vi "Resistive card.vi"(8 "error in (no error)":errorcluster, 11 "Node Ptr":T2 format="%.0x") -> (0 "error out":errorcluster)   [LabVIEW 2014, in "SLSC configuration System Explorer.lvlib"]
uses:
  SLSC configuration System Explorer.lvlib
  <vilib>/NI Veristand/Custom Device API/Custom Device Item Ref.ctl
  Shared/Card Postion.ctl
  Shared/Constants.vi
  <vilib>/NI Veristand/Custom Device API/Get Item Property (U16).vi
  <vilib>/NI Veristand/Custom Device API/Set Item Property (Variant).vi
  <vilib>/NI Veristand/Custom Device API/Custom Device API.lvlib
  Shared/SLSC configuration Shared.lvlib
panel:
  in  "Card Position":T1
  in  "CH 7 (ohms)":dbl min=0.0 max=8191.875 step=0.125 format="%#_7g"
  in  "CH 6 (ohms)":dbl min=0.0 max=8191.875 step=0.125 format="%#_7g"
  in  "CH 5 (ohms)":dbl min=0.0 max=8191.875 step=0.125 format="%#_7g"
  in  "CH 4 (ohms)":dbl min=0.0 max=8191.875 step=0.125 format="%#_7g"
  in  "CH 3(ohms)":dbl min=0.0 max=8191.875 step=0.125 format="%#_7g"
  in  "CH 2 (ohms)":dbl min=0.0 max=8191.875 step=0.125 format="%#_7g"
  in  "CH 1(ohms)":dbl min=0.0 max=8191.875 step=0.125 format="%#_7g"
  in  "Header 2":cluster{"Section Name":string}={"Section Name"="FIU Initial Configuration"}
  in  "CH 0 (ohms)":dbl min=0.0 max=8191.875 step=0.125 format="%#_7g"
  in  "Header":cluster{"Section Name":string}={"Section Name"="FIU Card Settings"}
  in  "Description":string
  in  "Name":string
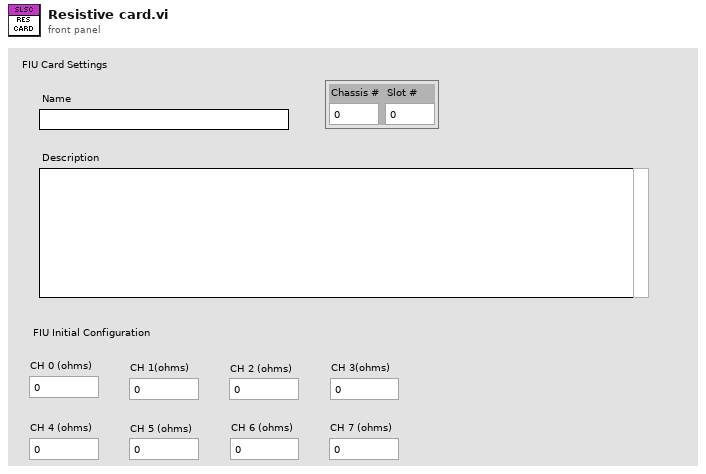
[diagram p1: front panel]
types:
  T1 = typedef "SLSC configuration Shared.lvlib/Card Postion.ctl" = cluster{"Chassis #":u8, "Slot #":u8}
  T2 = typedef "Custom Device API.lvlib/Custom Device Item Ref.ctl" = u64
  T3 = typedef "Custom Device API.lvlib/Custom Device Commands.ctl" = enum16{"Default", "Item renamed", "Shutdown", "Dynamic button pressed"}
  T4 = typedef "Custom Device API.lvlib/Custom Device Item Info.ctl" = cluster{"Name":string, "Is Channel":bool, "GUID":string, "Is Waveform":bool}
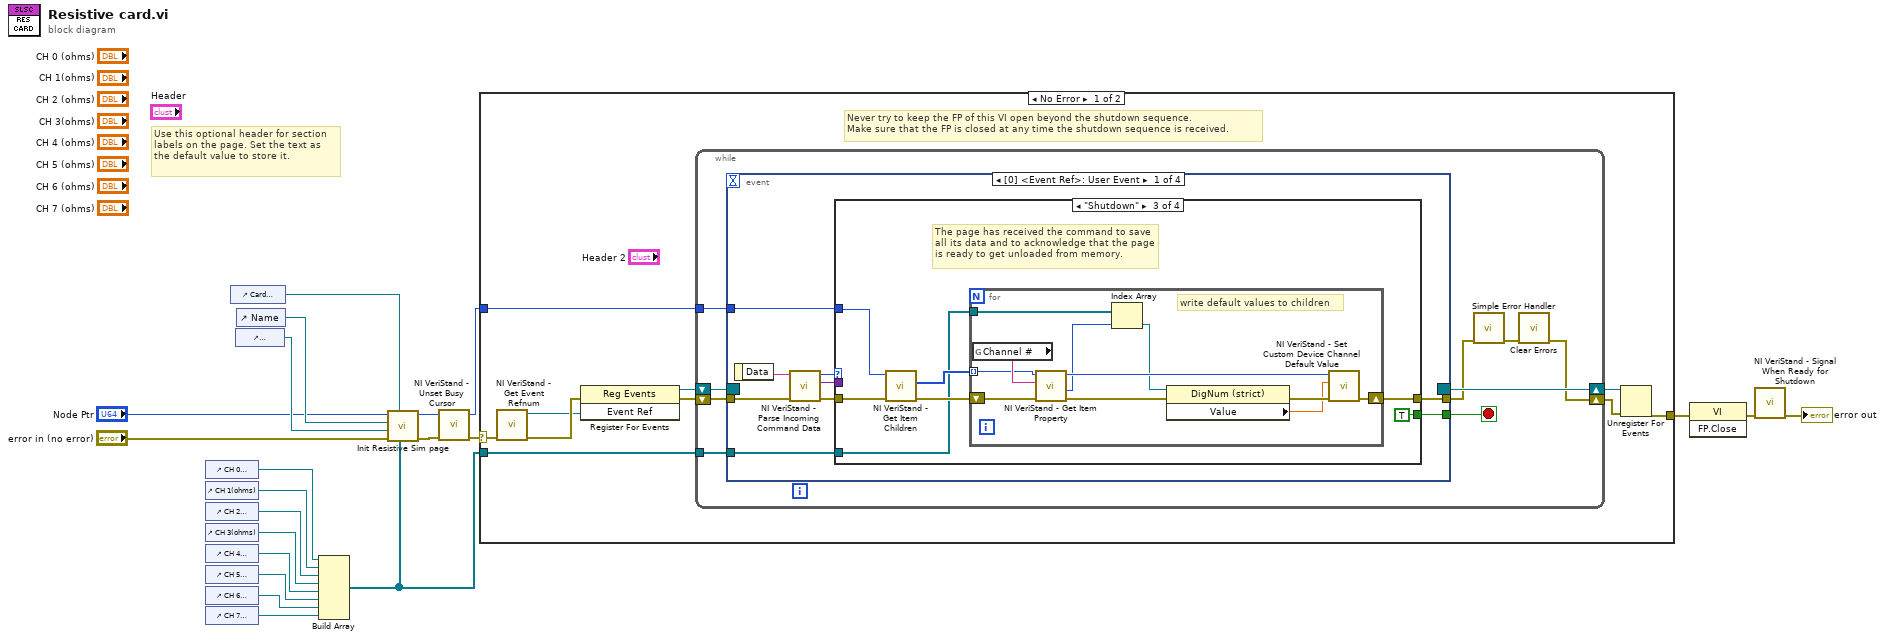
[diagram p0: block diagram]
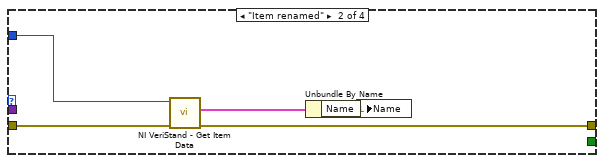
[diagram p3: hidden frame]
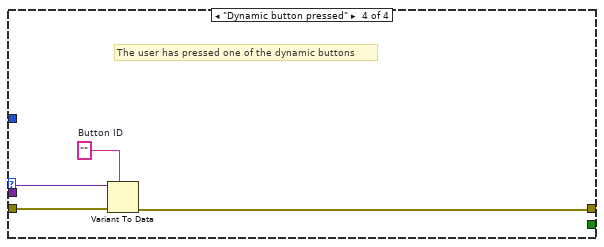
[diagram p4: hidden frame]
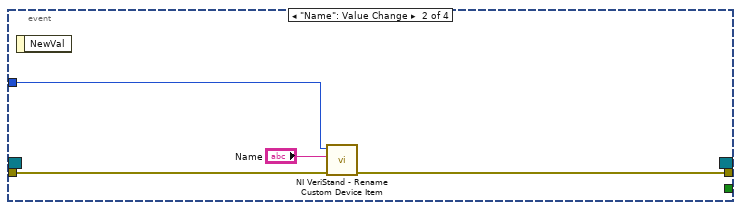
[diagram p5: hidden frame]
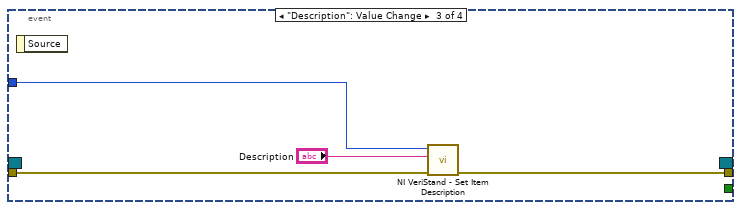
[diagram p6: hidden frame]
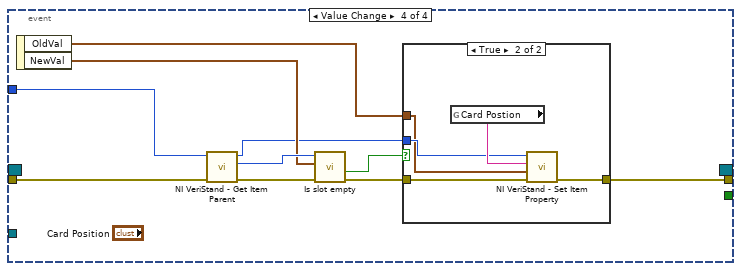
[diagram p7: hidden frame]
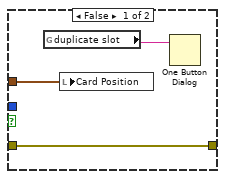
[diagram p8: hidden frame]
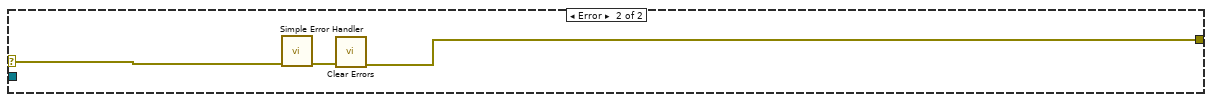
[diagram p9: hidden frame]
diagram:
  # "Use this optional header for section labels on the page. Set the text as the default value to store it."
  n1 = control-ref of="CH 0 (ohms)"() -> (w13:refnum<vi>)
  n2 = control-ref of="CH 1(ohms)"() -> (w12:refnum<vi>)
  n3 = control-ref of="CH 2 (ohms)"() -> (w11:refnum<vi>)
  n4 = control-ref of="CH 3(ohms)"() -> (w10:refnum<vi>)
  n5 = control-ref of="CH 4 (ohms)"() -> (w9:refnum<vi>)
  n6 = control-ref of="CH 5 (ohms)"() -> (w8:refnum<vi>)
  n7 = control-ref of="CH 6 (ohms)"() -> (w7:refnum<vi>)
  n8 = control-ref of="CH 7 (ohms)"() -> (w6:refnum<vi>)
  n9 = control-ref of="Card Position"() -> (w2:refnum<vi>)
  n10 = control-ref of="Description"() -> (w4:refnum<vi>)
  n11 = control-ref of="Name"() -> (w5:refnum<vi>)
  n12 = Build Array(w13, w12, w11, w10, w9, w8, w7, w6) -> (w3:refnum<vi>[])
  n13 = call "Init Resistive Sim page.vi"("Resistive sim controls"=w3, "Card Position"=w2, "error in (no error)"="error in (no error)", "Description"=w4, "Name"=w5, "Node Ptr"="Node Ptr") -> ("error out"=w17:errorcluster, "Node Ptr out"=w14:T2)  [unwired: 4 in]
  n14 = call <vilib>:"NI VeriStand - Unset Busy Cursor.vi"("error in (no error)"=w17) -> ("error out"=w16:errorcluster)  [unwired: 10 out]
  n15 = case shown="No Error" w16 {
    selector: w16 -> [w22 w105]
    tunnel: [w27 w103] -> w20
    tunnel: w14 -> [w23 _]
    tunnel: w3 -> [w21 _]
    frame No Error {
      # "Never try to keep the FP of this VI open beyond the shutdown sequence.\nMake sure that the FP is closed at any time the shutdown sequence is received."
      n16 = call <vilib>:"NI VeriStand - Get Event Refnum.vi"("error in (no error)"=w22) -> ("error out"=w30:errorcluster, "Event Ref"=w26:refnum<user-event>)  [unwired: 9 out]
      n17 = register-events(error in=w30, w26) -> (reference out=w24:refnum<event-registration>, error out=w25:errorcluster)  [unwired: 1 in]
      n18 = while {
        tunnel: w23 -> [w35]
        shift-right: [w32] -> w28
        shift-left: w25 -> [w38]
        shift-right: [w39] -> w29
        shift-left: w24 -> [w37]
        tunnel: w21 -> [w31]
        stop <- w36 stop-if-true
        n19 = event shown="[0] <Event Ref>: User Event" {
          selector: w37 -> [_ _ _ _]
          dyn-events: [_ _ _ _] -> w39
          timeout: _ -> [_ _ _ _]
          tunnel: w38 -> [w48 w80 w83 w86]
          tunnel: [w44 _ _ _] -> w36
          tunnel: [w43 w79 w82 w92] -> w34
          tunnel: w35 -> [w42 w78 w84 w91]
          tunnel: w31 -> [w40 _ _ _]
          event User Event {
            n20 = event-data() -> ("Data"=w47:string)  [unwired: 1 out]
            n21 = call <vilib>:"NI VeriStand - Parse Incoming Command Data.vi"("error in (no error)"=w48, "Incoming data"=w47) -> ("error out"=w46:errorcluster, "Outgoing data"=w41:variant, "Action"=w45:T3)  [unwired: 7 out]
            n22 = case shown="\"Shutdown\"" w45 {
              tunnel: w46 -> [w49 w54 w58 w76]
              tunnel: [_ _ TRUE _] -> w44
              tunnel: [w49 w51 w60 w73] -> w43
              tunnel: w42 -> [_ w53 w56 _]
              tunnel: w41 -> [_ _ _ w75]
              tunnel: w40 -> [_ _ w55 _]
              frame "Default", Default {
              }
              frame "Item renamed" {
                n23 = call <vilib>:"NI VeriStand - Get Item Data.vi"("error in (no error)"=w54, "Item Ref in"=w53) -> ("error out"=w51:errorcluster, "Item Info"=w52:T4)  [unwired: 8 out]
                n24 = Unbundle By Name(w52) -> ("Name"=w50:string)
                n25 = local write "Name"(w50) -> ()
              }
              frame "Shutdown" {
                # "The page has received the command to save all its data and to acknowledge that the page is ready to get unloaded from memory."
                n26 = call <vilib>:"NI VeriStand - Get Item Children.vi"("error in (no error)"=w58, "Item Ref in"=w56) -> ("error out"=w57:errorcluster, "Child Refs"=w59:T2[])  [unwired: 6 in, 2 out]
                n27 = for {
                  shift-right: [w70] -> w60
                  shift-left: w57 -> [w71]
                  tunnel: w59 -> [w66] mode=indexing
                  tunnel: w55 -> [w65]
                  # "write default values to children"
                  n28 = global read "Constants.vi" "Channel #"() -> (w72:string)
                  n29 = call-poly <vilib>:"NI VeriStand - Get Item Property.vi"("error in (no error)"=w71, "Property Name"=w72, "Item Ref in"=w66) -> ("error out"=w68:errorcluster, "Value"=w62:u16, "Item Ref out"=w69:T2)  [unwired: 5 in, 1 out]
                  n30 = Index Array(array=w65, index=w62) -> (element=w64:refnum<vi>)
                  n31 = property class="DigNum (strict)"(reference=w64, error in=w68) -> (error out=w67:errorcluster, "Value"=w63:dbl)  [unwired: 1 out]
                  n32 = call <vilib>:"NI VeriStand - Set Custom Device Channel Default Value.vi"("error in (no error)"=w67, "Default Value"=w63, "Channel Ref in"=w69) -> ("error out"=w70:errorcluster)  [unwired: 7 in, 1 out]
                }
              }
              frame "Dynamic button pressed" {
                w74 = ""  # Button ID
                # "The user has pressed one of the dynamic buttons"
                n33 = Variant To Data(error in=w76, type=w74, Variant=w75) -> (error out=w73:errorcluster)  [unwired: 1 out]
              }
            }
          }
          event "Name": Value Change {
            n34 = event-data() -> ()  [unwired: 2 out]
            n35 = call <vilib>:"NI VeriStand - Rename Custom Device Item.vi"("error in (no error)"=w80, "New Name"="Name", "Item Ref in"=w78) -> ("error out"=w79:errorcluster)  [unwired: 1 in, 7 out]
          }
          event "Description": Value Change {
            n36 = event-data() -> ()  [unwired: 2 out]
            n37 = call <vilib>:"NI VeriStand - Set Item Description.vi"("error in (no error)"=w83, "Description"="Description", "Item Ref in"=w84) -> ("error out"=w82:errorcluster)  [unwired: 8 out]
          }
          event Value Change {
            n38 = event-data() -> ("OldVal"=w85:T1, "NewVal"=w89:T1)  [unwired: 1 out]
            n39 = call <vilib>:"NI VeriStand - Get Item Parent.vi"("error in (no error)"=w86, "Item Ref in"=w91) -> ("error out"=w88:errorcluster, "Parent Ref"=w90:T2, "Item Ref out"=w87:T2)  [unwired: 6 in, 1 out]
            n40 = call "Is slot empty.vi"("error in (no error)"=w88, "Card Position"=w89, "Node Ptr"=w90) -> ("error out"=w94:errorcluster, "Empty?"=w93:bool)  [unwired: 6 in, 1 out]
            n41 = case shown="True" w93 {
              tunnel: w94 -> [w96 w99]
              tunnel: [w96 w101] -> w92
              tunnel: w87 -> [_ w100]
              tunnel: w85 -> [w95 w98]
              frame False {
                n42 = global read "Constants.vi" "duplicate slot"() -> (w97:string)
                n43 = local write "Card Position"(w95) -> ()
                n44 = One Button Dialog(message=w97) -> ()  [unwired: 1 in, 1 out]
              }
              frame True {
                n45 = global read "Constants.vi" "Card Postion"() -> (w102:string)
                n46 = call-poly <vilib>:"NI VeriStand - Set Item Property.vi"("error in (no error)"=w99, "Value"=w98, "Property Name"=w102, "Item Ref in"=w100) -> ("error out"=w101:errorcluster)  [unwired: 5 in, 2 out]
              }
            }
          }
        }
        n47 = call <vilib>:"Simple Error Handler.vi"("error in (no error)"=w34) -> ("error out"=w33:errorcluster)  [unwired: 1 in, 7 out]
        n48 = call <vilib>:"Clear Errors.vi"("error in (no error)"=w33) -> ("error out"=w32:errorcluster)  [unwired: 1 in, 5 out]
      }
      n49 = Unregister For Events(event registration refnum=w29, error in=w28) -> (error out=w27:errorcluster)
    }
    frame Error {
      n50 = call <vilib>:"Simple Error Handler.vi"("error in (no error)"=w105) -> ("error out"=w104:errorcluster)  [unwired: 1 in, 7 out]
      n51 = call <vilib>:"Clear Errors.vi"("error in (no error)"=w104) -> ("error out"=w103:errorcluster)  [unwired: 1 in, 5 out]
    }
  }
  n52 = invoke class="VI" method="FP.Close"(error in=w20) -> (error out=w19:errorcluster)  [unwired: 2 in, 2 out]
  n53 = call <vilib>:"NI VeriStand - Signal When Ready for Shutdown.vi"("error in (no error)"=w19) -> ("error out"=→"error out":errorcluster)  [unwired: 10 out]
